vi "assoc.vi"(11 "input 1":string) -> (3 "standard output":string)   [LabVIEW 2014]
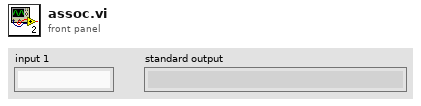
[diagram p1: front panel]
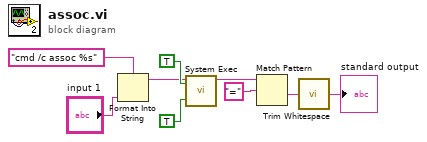
[diagram p0: block diagram]
diagram:
  n1 = Format Into String(format string="cmd /c assoc %s" ("command line"), "input 1") -> (resulting string=w2:string)  [unwired: 2 in, 1 out]
  n2 = call <vilib>:"System Exec.vi"("run minimized? (F)"=TRUE, "wait until completion? (T)"=TRUE, "command line"=w2) -> ("standard output"=w7:string)  [unwired: 5 in, 3 out]
  n3 = Match Pattern(string=w7, regular expression="=") -> (after substring=w9:string)  [unwired: 1 in, 3 out]
  n4 = call <vilib>:"Trim Whitespace.vi"("string"=w9) -> ("trimmed string"=→"standard output":string)  [unwired: 1 in]
